vi "Write_Instr.vi"(8 "error in (no error)":errorcluster caption="entrée d'erreur (pas d'erreur)", 11 "Class Relay_Board en entrée":refnum<class "Class Instrument Relay_Board.lvclass">) -> (0 "error out":errorcluster caption="sortie d'erreur", 3 "Class Relay_Board en Sortie":refnum<class "Class Instrument Relay_Board.lvclass">)   [LabVIEW 2020, in "Library Instrument & Equipement.lvlib" / "Library Instruments.lvlib" / "Class Instrument Relay_Board.lvclass"]
uses:
  Class Instrument Relay_Board.lvclass
  Class Instrument Relay_Board.lvclass/Class Instrument Relay_Board.ctl
  Instrument (Default)/Class Instrument (Default).lvclass
  Relay_Board/Relay_Board (Default)/Class Relay_Board (Default).lvclass
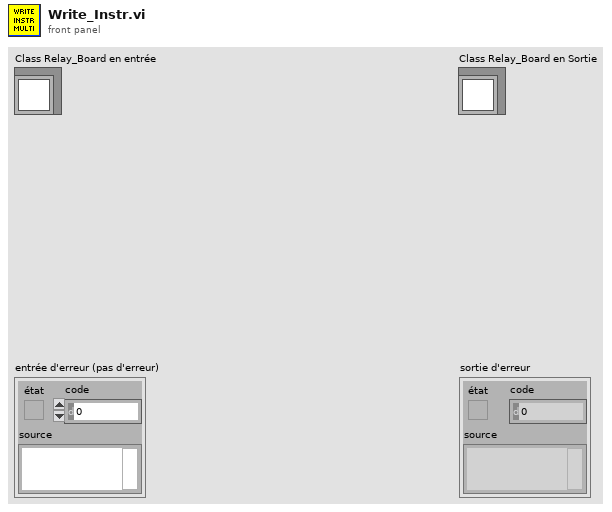
[diagram p1: front panel]
types:
  T1 = typedef "Library Commun.lvlib/Data_Write_Relay_Board.ctl" = enum16{"Enable Relays", "Disable Relays"}
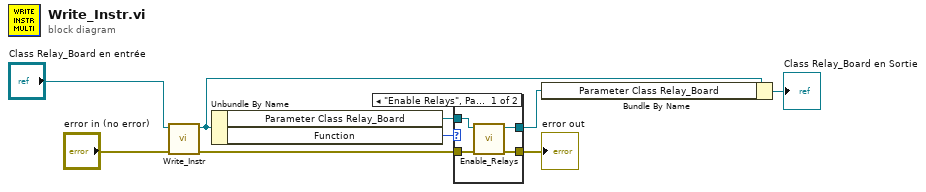
[diagram p0: block diagram]
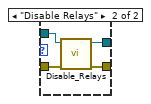
[diagram p2: hidden frame]
diagram:
  n1 = call-parent "Write_Instr.vi"("error in (no error)"="error in (no error)", "Class Multimeter (Default) en entrée"="Class Relay_Board en entrée") -> ("error out"=w6:errorcluster, "Class Multimeter (Default) en sortie"=w2:refnum<class "Class Instrument Relay_Board.lvclass">)  [unwired: 8 in]
  n2 = Unbundle By Name(w2) -> ("Parameter Class Relay_Board"=w4:refnum<class "Class Relay_Board (Default).lvclass">, "Function"=w7:T1)
  n3 = case shown="\"Enable Relays\", Par défaut" w7 {
    tunnel: w6 -> [w13 w17]
    tunnel: [w12 w16] -> w5
    tunnel: w4 -> [w11 w15]
    tunnel: [w10 w14] -> w3
    frame "Enable Relays", Default {
      n4 = call-dynamic "Enable_Relays.vi"("error in (no error)"=w13, "Class Relay_Board (Default) en entrée"=w11) -> ("error out"=w12:errorcluster, "Class Relay_Board (Default) en sortie"=w10:refnum<class "Class Relay_Board (Default).lvclass">)  [unwired: 8 in]
    }
    frame "Disable Relays" {
      n5 = call-dynamic "Disable_Relays.vi"("error in (no error)"=w17, "Class Relay_Board (Default) en entrée"=w15) -> ("error out"=w16:errorcluster, "Class Relay_Board (Default) en sortie"=w14:refnum<class "Class Relay_Board (Default).lvclass">)  [unwired: 8 in]
    }
  }
  "error out" <- w5
  n6 = Bundle By Name(cluster=w2, "Parameter Class Relay_Board"=w3) -> (→"Class Relay_Board en Sortie":refnum<class "Class Instrument Relay_Board.lvclass">)
